vi "Xively.vi"() -> ()   [LabVIEW 2011]
uses:
  <vilib>/httpClient/LabVIEWHTTPClient.lvlib
panel:
  out "Temperature":u8(slide) scale=0.0..100.0
  in  "?":bool
  out "Elapsed Time (s)":dbl
  out "Feed":bool caption="Time has Elapsed"
  in  "API Key":string="Vxd8EgTVhReb77kQqLWyJVSu0nNxgQ4AHZjfj17twepAdGTq"
  in  "Feed ID":string="58546256"
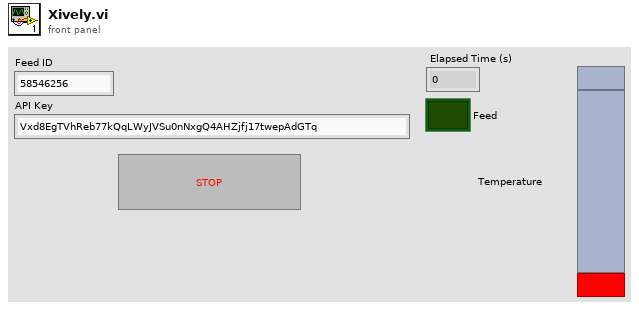
[diagram p1: front panel]
types:
  T1 = typedef "LabVIEWHTTPClient.lvlib/ClientHandle.ctl" = refnum<k1>
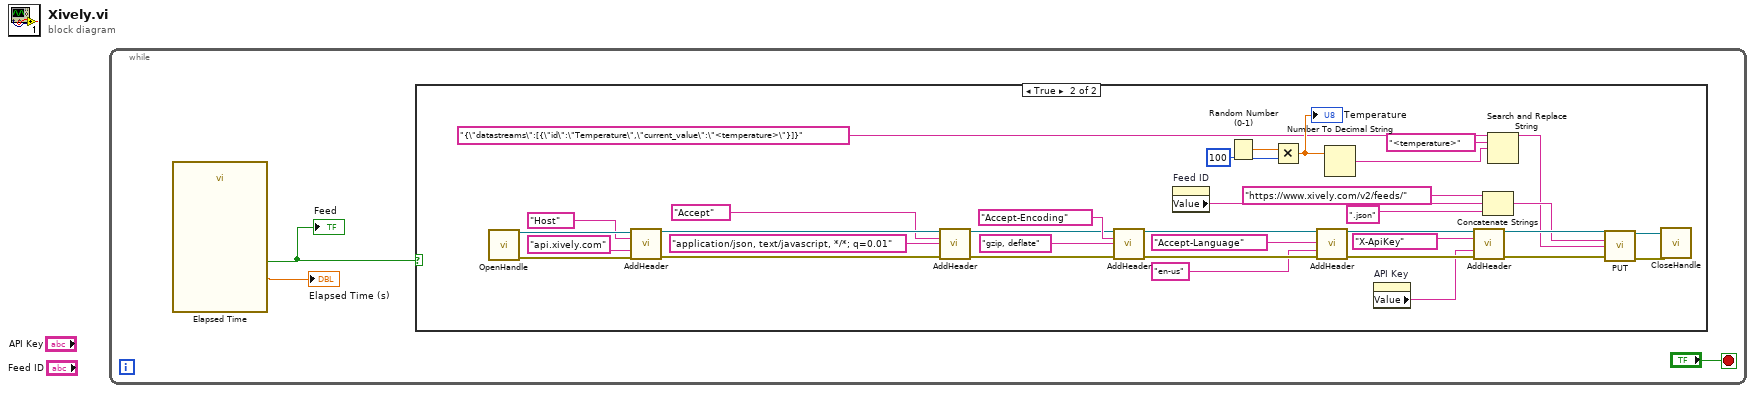
[diagram p0: block diagram]
diagram:
  n1 = while {
    stop <- "?" stop-if-true
    n2 = call "Elapsed Time"() -> ("Elapsed Time (s)"=→"Elapsed Time (s)":dbl, "Time has Elapsed"=w2:bool)  [unwired: 12 in, 6 out]
    "Feed" <- w2
    n3 = case shown="True" w2 {
      frame False {
      }
      frame True {
        n4 = call <vilib>:"OpenHandle.vi"() -> ("client handle out"=w31:T1, "error out"=w30:errorcluster)  [unwired: 14 in]
        n5 = call <vilib>:"AddHeader.vi"("client handle"=w31, "header"="Host", "value"="api.xively.com", "error in (no error)"=w30) -> ("client handle out"=w27:T1, "error out"=w26:errorcluster)  [unwired: 10 in]
        n6 = call <vilib>:"AddHeader.vi"("client handle"=w27, "header"="Accept", "value"="application/json, text/javascript, */*; q=0.01", "error in (no error)"=w26) -> ("client handle out"=w22:T1, "error out"=w21:errorcluster)  [unwired: 10 in]
        n7 = call <vilib>:"AddHeader.vi"("client handle"=w22, "header"="Accept-Encoding", "value"="gzip, deflate", "error in (no error)"=w21) -> ("client handle out"=w19:T1, "error out"=w18:errorcluster)  [unwired: 10 in]
        n8 = property on="Feed ID" class="Str"() -> ("Value"=w4:string)  [unwired: 2 in, 2 out]
        n9 = Random Number (0-1)() -> (number: 0 to 1=w35:dbl)
        n10 = Multiply(x=w35, y=100) -> (x*y=w37:dbl)
        "Temperature" <- w37
        n11 = call <vilib>:"AddHeader.vi"("client handle"=w19, "header"="Accept-Language", "value"="en-us", "error in (no error)"=w18) -> ("client handle out"=w15:T1, "error out"=w14:errorcluster)  [unwired: 10 in]
        n12 = Number To Decimal String(number=w37) -> (decimal integer string=w12:string)  [unwired: 1 in]
        n13 = property on="API Key" class="Str"() -> ("Value"=w5:string)  [unwired: 2 in, 2 out]
        n14 = call <vilib>:"AddHeader.vi"("client handle"=w15, "header"="X-ApiKey", "value"=w5, "error in (no error)"=w14) -> ("client handle out"=w34:T1, "error out"=w33:errorcluster)  [unwired: 10 in]
        n15 = Concatenate Strings("https://www.xively.com/v2/feeds/" ("url"), w4, ".json" ("string")) -> (w9:string)
        n16 = Search and Replace String(input string="{\"datastreams\":[{\"id\":\"Temperature\",\"current_value\":\"<temperature>\"}]}", search string="<temperature>", replace string=w12) -> (result string=w8:string)  [unwired: 5 in, 3 out]
        n17 = call <vilib>:"PUT.vi"("client handle"=w34, "url"=w9, "data"=w8, "error in (no error)"=w33) -> ("client handle out"=w7:T1, "error out"=w6:errorcluster)  [unwired: 8 in, 2 out]
        n18 = call <vilib>:"CloseHandle.vi"("client handle"=w7, "error in (no error)"=w6) -> ()  [unwired: 13 in, 1 out]
      }
    }
  }
